vi "H.Signal.vi"() -> (4 "output cluster":T1, 10 "Error Message":string, 13 "Camera & LVDT cyl":T2, 15 "Bool_H Sig":bool)   [LabVIEW 2015]
uses:
  Galobal variable_TI.vi
panel:
  in  "Cluster":T1
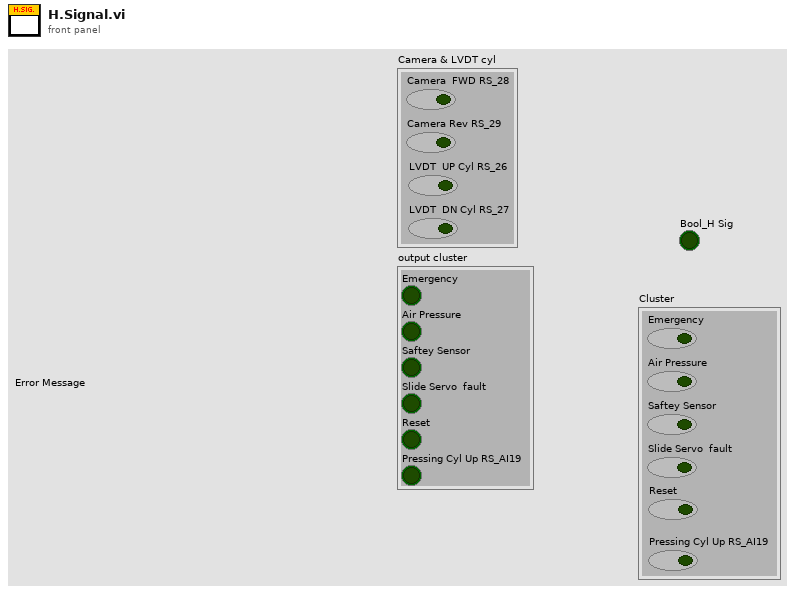
[diagram p1: front panel]
types:
  T1 = cluster{"Emergency":bool, "Air Pressure":bool, "Saftey Sensor":bool, "Slide Servo  fault":bool, "Reset":bool, "Pressing Cyl Up RS_AI19":bool}
  T2 = cluster{"Camera  FWD RS_28":bool, "Camera Rev RS_29":bool, "LVDT  UP Cyl RS_26":bool, "LVDT  DN Cyl RS_27":bool}
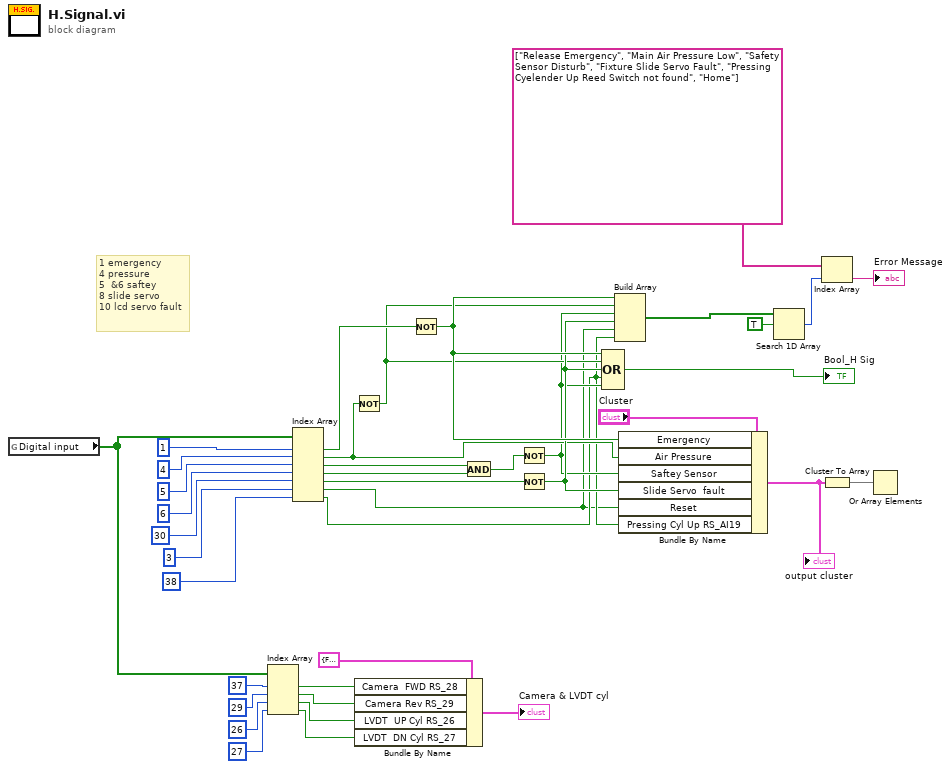
[diagram p0: block diagram]
diagram:
  # "1 emergency\n4 pressure\n5  &6 saftey\n8 slide servo\n10 lcd servo fault"
  n1 = global read "Galobal variable_TI.vi" "Digital input"() -> (w15:bool[])
  n2 = Index Array(array=w15, index #1=37 ("index"), index #2=29 ("index"), index #3=26 ("index"), index #4=27 ("index")) -> (element #1=w11:bool, element #2=w10:bool, element #3=w7:bool, element #4=w6:bool)
  n3 = Index Array(array=w15, index #1=1 ("index"), index #2=4 ("index"), index #3=5 ("index"), index #4=6 ("index"), index #5=30 ("index"), index #6=3 ("index"), index #7=38 ("index")) -> (element #1=w24:bool, element #2=w18:bool, element #3=w4:bool, element #4=w33:bool, element #5=w22:bool, element #6=w1:bool, element #7=w2:bool)
  n4 = Not(x=w18) -> (.not. x?=w17:bool)
  n5 = Bundle By Name(cluster=T2 {"Camera  FWD RS_28"=FALSE, "Camera Rev RS_29"=FALSE, "LVDT  UP Cyl RS_26"=FALSE, "LVDT  DN Cyl RS_27"=FALSE} ("Camera & LVDT cyl"), "Camera  FWD RS_28"=w11, "Camera Rev RS_29"=w10, "LVDT  UP Cyl RS_26"=w7, "LVDT  DN Cyl RS_27"=w6) -> (→"Camera & LVDT cyl":T2)
  n6 = Not(x=w24) -> (.not. x?=w20:bool)
  n7 = And(x=w4, y=w33) -> (x .and. y?=w23:bool)
  n8 = Not(x=w23) -> (.not. x?=w16:bool)
  n9 = Not(x=w22) -> (.not. x?=w19:bool)
  n10 = Compound Arithmetic op=OR(w20, w17, w19, w2, w16) -> (→"Bool_H Sig":bool)
  n11 = Build Array(w20, w17, w16, w19, w1, w2) -> (w29:bool[])
  n12 = Bundle By Name(cluster="Cluster", "Emergency"=w20, "Air Pressure"=w18, "Saftey Sensor"=w16, "Slide Servo  fault"=w19, "Reset"=w1, "Pressing Cyl Up RS_AI19"=w2) -> (w28:T1)
  "output cluster" <- w28
  n13 = Search 1D Array(1D array=w29, element=TRUE) -> (index of element=w31:i32)  [unwired: 1 in]
  n14 = Index Array(array=string[] ["Release Emergency", "Main Air Pressure Low", "Safety Sensor Disturb", "Fixture Slide Servo Fault", "Pressing Cyelender Up Reed Switch not found", "Home"], index=w31) -> (element=→"Error Message":string)
  n15 = Cluster To Array(cluster=w28) -> (array=w27:bool[])
  n16 = Or Array Elements(Boolean array=w27) -> ()  [unwired: 1 out]
